vi "state control module.vi"(9 "results in":T2, 10 "parameters in":T2, 11 "state control in":T1) -> (1 "results out":T2, 2 "parameters out":T2, 3 "state control out":T1)   [LabVIEW 2013, in "configuration tests.lvlib" / "TEST RUNTIME.lvclass"]
uses:
  TEST RUNTIME.lvclass
  <vilib>/NI/Tag Bus/table/data table.ctl
  state control.ctl
  <vilib>/NI/Tag Bus/table/data polymorphs/read one/read Double.vi
  <vilib>/NI/Tag Bus/table/data polymorphs/write one/write Double.vi
  <vilib>/NI/Tag Bus/table/data table.lvlib
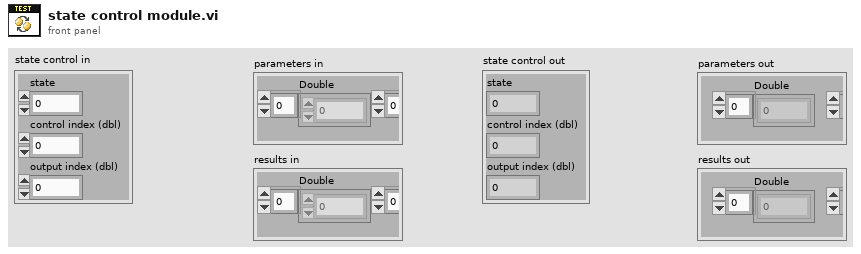
[diagram p1: front panel]
types:
  T1 = typedef "configuration tests.lvlib/TEST RUNTIME.lvclass/state control.ctl" = cluster{"state":u8, "control index (dbl)":i32, "output index (dbl)":i32}
  T2 = typedef "tag bus.lvlib/data table.lvlib/data table.ctl" = cluster{"Double":dbl[], "Single":sgl[], "I64":i64[], "I32":i32[], "I16":i16[], "I8":i8[], "U64":u64[], "U32":u32[], "U16":u16[], "U8":u8[], "Boolean":bool[], "String":string[], "Array of Double":cluster{"DBL Array":dbl[]}[], "Array of Single":cluster{"SGL Array":sgl[]}[], "Array of I64":cluster{"I64 Array":i64[]}[], "Array of I32":cluster{"I32 Array":i32[]}[], "Array of I16":cluster{"I16 Array":i16[]}[], "Array of I8":cluster{"I8 Array":i8[]}[], "Array of U64":cluster{"U64 Array":u64[]}[], "Array of U32":cluster{"U32 Array":u32[]}[], "Array of U16":cluster{"U16 Array":u16[]}[], "Array of U8":cluster{"U8 Array":u8[]}[], "Array of Boolean":cluster{"Boolean Array":bool[]}[], "Array of String":cluster{"String Array":string[]}[]}
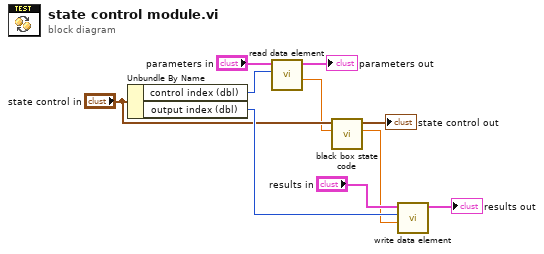
[diagram p0: block diagram]
diagram:
  n1 = Unbundle By Name("state control in") -> ("control index (dbl)"=w6:i32, "output index (dbl)"=w5:i32)
  n2 = call-poly <vilib>:"read data element.vi"("index"=w6, "data table in"="parameters in") -> ("value"=w1:dbl, "data table out"=→"parameters out":T2)  [unwired: 8 in]
  n3 = call "black box state code.vi"("value in"=w1, "state control in"="state control in") -> ("value out"=w3:dbl, "state control out"=→"state control out":T1)  [unwired: 8 in]
  n4 = call-poly <vilib>:"write data element.vi"("value"=w3, "index"=w5, "data table in"="results in") -> ("data table out"=→"results out":T2)  [unwired: 8 in]
